vi "TestElevatorPID.vi"() -> ()   [LabVIEW 2018]
uses:
  <vilib>/Rock Robotics/WPI/ThirdParty/REV Robotics/SPARK MAX/Typedef/Spark MAX Control Type.ctl
panel:
  in  "stop":bool
  out "Waveform Chart":cluster{"Setpoint":dbl, "Sensor Position":dbl}(graph)
  in  "Setpoint":dbl
  in  "PID Constants":T1={"P Gain"=0.0, "I Gain"=0.0, "D Gain"=0.0, "F Gain"=0.0, "I Zone"=0.0, "Min Output"=-1.0, "Max Output"=1.0}
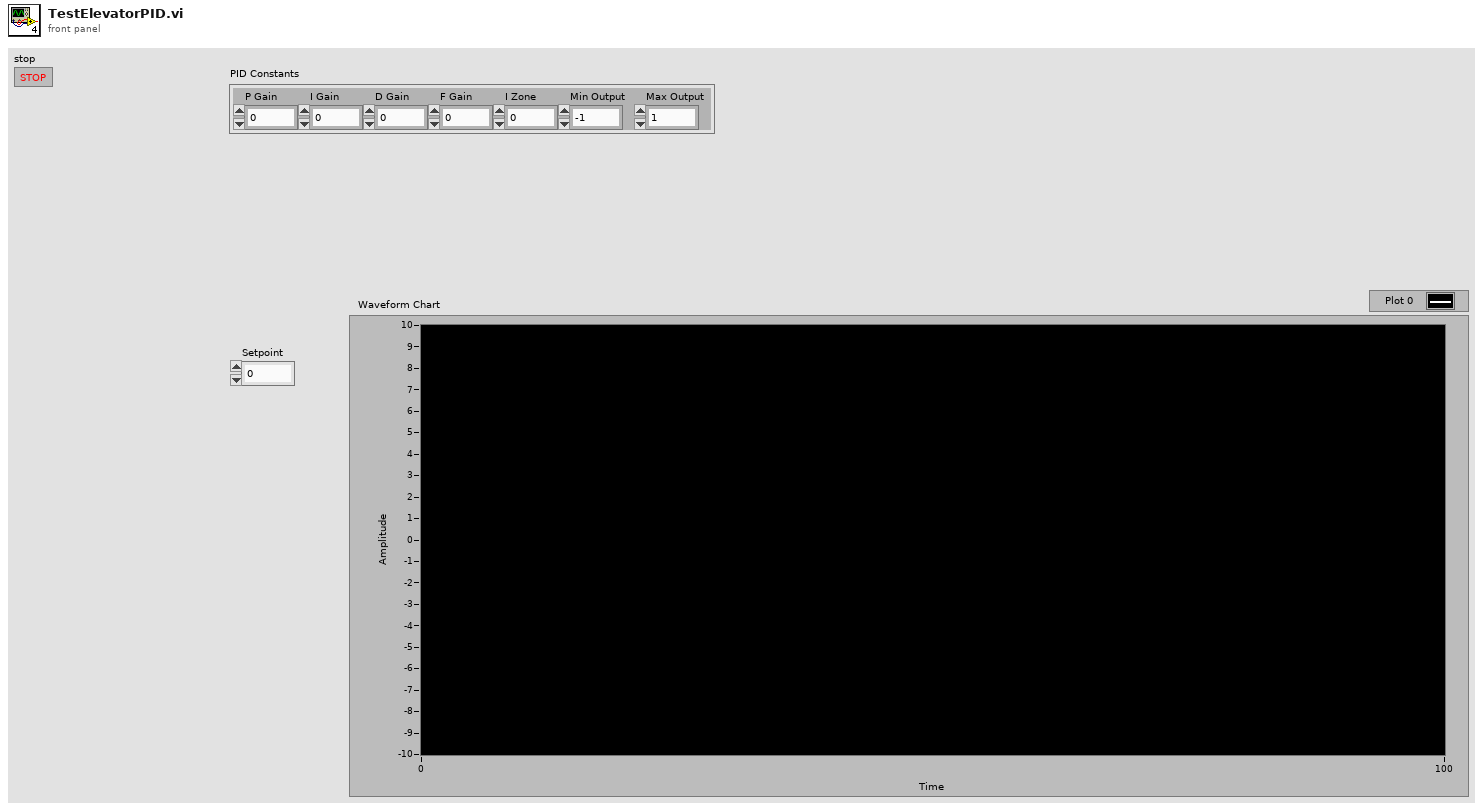
[diagram p1: front panel]
types:
  T1 = cluster{"P Gain":dbl, "I Gain":dbl, "D Gain":dbl, "F Gain":dbl, "I Zone":dbl, "Min Output":dbl, "Max Output":dbl}
  T2 = typedef "WPI_MotorControlDeviceRef.ctl" = cluster{"DeviceStatus":errorcluster, "Type":T3, "PWM":cluster{"PWM Channel":T4, "DeadBand":T5}, "CAN":cluster{"Device Number":u8, "SetOutput VI Ref":variant, "GetOutput VI Ref":variant, "Enable VI Ref":variant, "Disable VI Ref":variant, "Data":variant}, "Invert":bool, "DIO PWM":cluster{"PWM \"Enable\" Channel":T4, "DIOChannel":T6, "PWM Rate":dbl}}
  T3 = typedef "WPI_MotorControlType.ctl" = enum16{"PWM", "CAN", "DIO PWM"}
  T4 = typedef "FPGA_DIOPWMChannel.ctl" = enum8{"PWM 0", "PWM 1", "PWM 2", "PWM 3", "PWM 4", "PWM 5", "PWM 6", "PWM 7", "PWM 8", "PWM 9", "PWM MXP 0", "PWM MXP 1", "PWM MXP 2", "PWM MXP 3", "PWM MXP 4", "PWM MXP 5", "PWM MXP 6", "PWM MXP 7", "PWM MXP 8", "PWM MXP 9", "Invalid"}
  T5 = typedef "WPI_PWMDeadband.ctl" = cluster{"Name":string, "maxPositivePwm":i32, "minPositivePwm":i32, "centerPwm":i32, "maxNegativePwm":i32, "minNegativePwm":i32, "angularRange":u16}
  T6 = typedef "FPGA_DIOChannel.ctl" = enum8{"DIO 0", "DIO 1", "DIO 2", "DIO 3", "DIO 4", "DIO 5", "DIO 6", "DIO 7", "DIO 8", "DIO 9", "DIO MXP 0", "DIO MXP 1", "DIO MXP 2", "DIO MXP 3", "DIO MXP 4", "DIO MXP 5", "DIO MXP 6", "DIO MXP 7", "DIO MXP 8", "DIO MXP 9", "DIO MXP 10", "DIO MXP 11", "DIO MXP 12", "DIO MXP 13", "DIO MXP 14", "DIO MXP 15", "SPI Port CS1", "SPI Port CS2", "SPI Port CS3", "SPI Port MISO", "SPI Port MOSI", "Invalid"}
  T7 = cluster{"P Gain":bool, "I Gain":bool, "D Gain":bool, "F Gain":bool, "I Zone":bool, "Min Output":bool, "Max Output":bool}
  T8 = typedef "Spark MAX Control Type.ctl" = enum16{"Percent VBus", "Voltage", "Velocity", "Position", "Smart Motion", "Current", "Smart Velocity"}
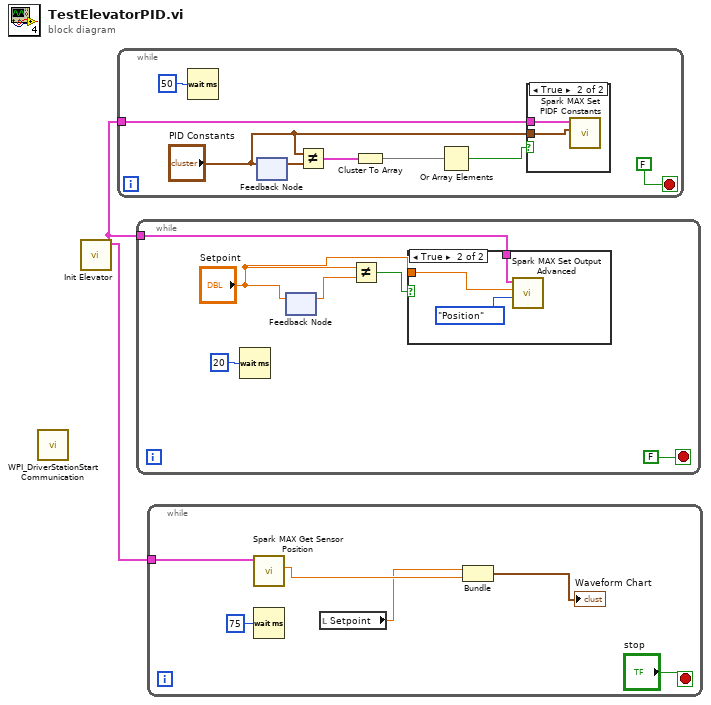
[diagram p0: block diagram]
diagram:
  n1 = call <vilib>:"WPI_DriverStationStart Communication.vi"() -> ()  [unwired: 12 in]
  n2 = call "Init Elevator.vi"() -> ("Master Out"=w1:T2)  [unwired: 10 in, 1 out]
  n3 = while {
    tunnel: w1 -> [w5]
    stop <- FALSE stop-if-true
    n4 = Wait (ms)(milliseconds to wait=u32 50) -> ()  [unwired: 1 out]
    n5 = feedback-in #1("PID Constants") -> ()
    n6 = feedback #1() -> (w9:T1)  [unwired: 1 in]
    n7 = Not Equal?(x="PID Constants", y=w9) -> (x != y?=w8:T7)
    n8 = Cluster To Array(cluster=w8) -> (array=w7:bool[])
    n9 = Or Array Elements(Boolean array=w7) -> (logical OR=w6:bool)
    n10 = case shown="True" w6 {
      tunnel: w5 -> [_ w11]
      tunnel: "PID Constants" -> [_ w10]
      frame False {
      }
      frame True {
        n11 = call <vilib>:"Spark MAX Set PIDF Constants.vi"("PID Constants"=w10, "MotorControlDeviceRef"=w11) -> ()  [unwired: 8 in, 2 out]
      }
    }
  }
  n12 = while {
    tunnel: w1 -> [w14]
    stop <- FALSE stop-if-true
    n13 = Wait (ms)(milliseconds to wait=u32 20) -> ()  [unwired: 1 out]
    n14 = feedback-in #2("Setpoint") -> ()
    n15 = feedback #2() -> (w17:dbl)  [unwired: 1 in]
    n16 = Not Equal?(x="Setpoint", y=w17) -> (x != y?=w13:bool)
    n17 = case shown="True" w13 {
      tunnel: w14 -> [_ w20]
      tunnel: "Setpoint" -> [_ w19]
      frame False {
      }
      frame True {
        n18 = call <vilib>:"Spark MAX Set Output Advanced.vi"("Control Mode"=Spark_MAX_Control_Type."Position", "Setpoint"=w19, "MotorControlDevRef"=w20) -> ()  [unwired: 7 in, 2 out]
      }
    }
  }
  n19 = while {
    tunnel: w1 -> [w25]
    stop <- "stop" stop-if-true
    n20 = call <vilib>:"Spark MAX Get Sensor Position.vi"("MotorControlDevRef in"=w25) -> ("Sensor Position"=w26:dbl)  [unwired: 7 in, 3 out]
    n21 = Wait (ms)(milliseconds to wait=u32 75) -> ()  [unwired: 1 out]
    n22 = local read "Setpoint"() -> (w24:dbl)
    n23 = Bundle("Setpoint"=w24, "Sensor Position"=w26) -> (→"Waveform Chart":cluster{"Setpoint":dbl, "Sensor Position":dbl})  [unwired: 1 in]
  }
